vi "BurstRecognition.vi"(2 "IntensityTrace":u32[](array[numeric]), 3 "Parameters":T1={"PeakThreshold"=40, "RecognitionThreshold"=20, "SeparationLimit"=0.7} {"SeparationLimit" format="%.2f"}) -> (0 "Index Hi":u32[](array[numeric]), 1 "Index Low":u32[](array[numeric]))   [LabVIEW 2009]
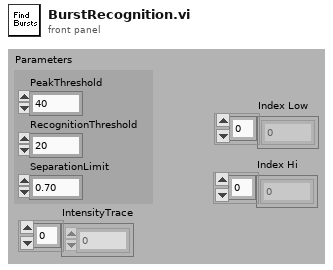
[diagram p1: front panel]
types:
  T1 = cluster{"PeakThreshold":u32, "RecognitionThreshold":u32, "SeparationLimit":sgl}
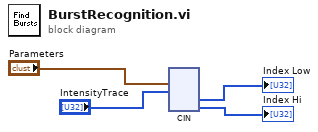
[diagram p0: block diagram]
diagram:
  n1 = cin("Parameters", "IntensityTrace") -> (→"Index Low":u32[], →"Index Hi":u32[])  [unwired: 4 in]
